vi "Functional acq video generator.vi"(7 "Channel":enum16{"Green", "Red"}(ring)=enum."Red", 9 "Input cluster":T2={"# of frames to export"=0, "Initial frame's owning file"=refnum, "8-bit AVI file path"=path "", "Cursors location"={"Number of first cycle"=0, "Number of last cycle"=100}}, 11 "ExperimentPath":path=path "C:/Users/Teo/Desktop/UCL Datasets/160915_13_48_57 FunctAcq-6 patches") -> ()   [LabVIEW 2020]
uses:
  Typedefs/Experiment Parameters.ctl
  Typedefs/Bright-Contr-Gamma cluster.ctl
  Timelapse Viewer/Typedefs/Speed graph behaviour enum.ctl
  <vilib>/vision/Avi.llb/IMAQ AVI2 Refnum.ctl
  Timelapse Viewer/Typedefs/8-bit video export window ctrl refs.ctl
  <vilib>/Utility/miscctls.llb/LVPointTypeDef.ctl
  Functional Imaging Viewer/Typedefs/Get-Set-Clear Control.ctl
  Timelapse Viewer/Globals/gl_Time series viewer globals.vi
  Globals/gl_8-bit montage window ctrl refs.vi
panel:
  in  "Speed graph behaviour":T3
  in  "Codec":u16(ring)=5 items=["No Codec", "Intel IYUV codec", "Cinepak Codec by Radius", "Microsoft Video 1", "FF Video Codec 1 (FFV1) (NI Vision)", "Motion JPEG (NI Vision)", "Y800 Uncompressed Grey Scale (NI Vision)", "YUV 4:2:0 Planar (NI Vision)"]
  in  "Microscope Image Adjustments":T4={"Brightness"=128.0, "Contrast"=45.0, "Gamma"=1.0} {"Gamma" min=0.5 scale=0.0..2.0; "Contrast" min=0.5 scale=0.0..90.0; "Brightness" min=0.5 scale=0.0..250.0}
  in  "Camera Video Adjustments":T4={"Brightness"=128.0, "Contrast"=45.0, "Gamma"=1.0} {"Gamma" min=0.5 scale=0.0..2.0; "Contrast" min=0.5 scale=0.0..90.0; "Brightness" min=0.5 scale=0.0..250.0}
  in  "Height of bottom tier":u32=120
  out "Frames Per Second":u32=26
  in  "Peak value in dataset (I16)":dbl=4000.0 format="%#_13g"
  in  "Number of rows to generate":i32=2
  in  "Execute":bool
  in  "Include speed graph":bool=TRUE
  in  "Include camera videos":bool
  in  "Enable saving":bool
  out "Image":T5(plugin-control)
  in  "Stop button":bool
  out "Global cycle number among all trials":i32 format="Current cycle: %.0f"
  out "Completion status":u8(slide) scale=0.0..100.0
  out "error out":errorcluster
  out "Experiment Parameters":T6
  out "Status":string
  # "This VI will be upgraded to handle volumetric data."
  # "<-- Adjusts the output dynamic range.\n       Temporary control."
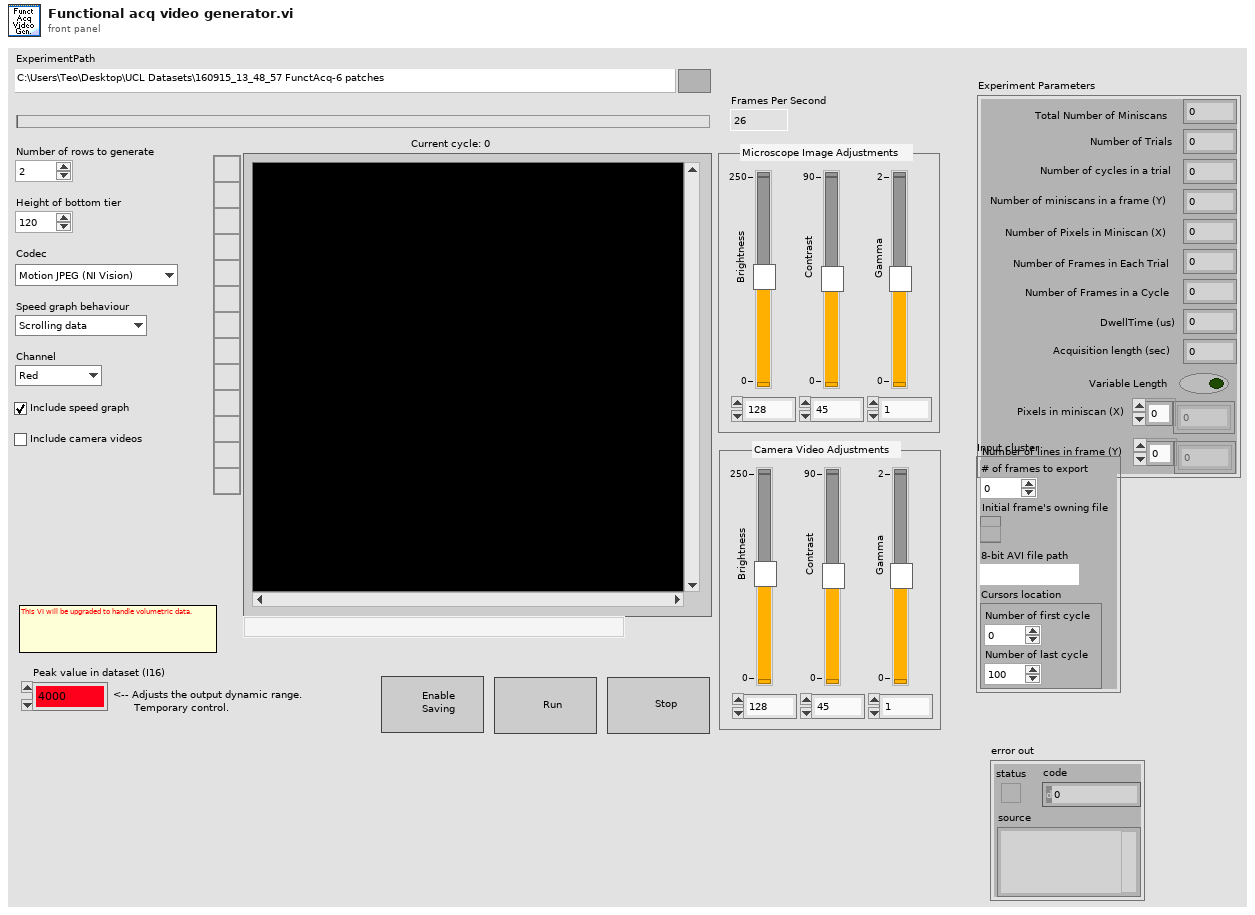
[diagram p1: front panel]
types:
  T1 = typedef "IMAQ AVI2 Refnum.ctl" = refnum<k20>
  T2 = cluster{"# of frames to export":i32, "Initial frame's owning file":T1, "8-bit AVI file path":path, "Cursors location":cluster{"Number of first cycle":i32, "Number of last cycle":i32}}
  T3 = typedef "Speed graph behaviour enum.ctl" = enum16{"Scrolling data", "Scrolling cursor"}
  T4 = typedef "Bright-Contr-Gamma cluster.ctl" = cluster{"Brightness":sgl, "Contrast":sgl, "Gamma":sgl}
  T5 = typedef "IMAQ Image.ctl" = refnum<image>
  T6 = typedef "Experiment Parameters.ctl" = cluster{"Total Number of Miniscans":i32, "Number of Trials":i32, "Number of cycles in a trial":i32, "Number of miniscans in a frame (Y)":i32, "Number of Pixels in Miniscan (X)":i32, "Number of Frames in Each Trial":i32, "Number of Frames in a Cycle":i32, "DwellTime (us)":dbl, "Acquisition length (sec)":dbl, "Variable Length":bool, "Pixels in miniscan (X)":dbl[], "Number of lines in frame (Y)":dbl[]}
  T7 = typedef "8-bit video export window ctrl refs.ctl" = cluster{"This VI":refnum<vi>, "Add speed data":refnum<vi>, "Add camera videos":refnum<vi>, "Stop button":refnum<vi>, "Camera Video Adjustments":refnum<vi>, "Microscope Image Adjustments":refnum<vi>, "Execute":refnum<vi>, "Codec":refnum<vi>, "Channel to load":refnum<vi>, "Speed graph behaviour":refnum<vi>, "Include speed graph":refnum<vi>, "Number of rows to generate":refnum<vi>, "Path":refnum<vi>}
  T8 = typedef "AVI playback header info cluster.ctl" = cluster{"Frame Size":u32, "AOD fill time (us)":dbl, "Dwell time (us)":dbl, "Frame period (ms)":dbl, "Number of Miniscans":u16, "Number of Pixels in Miniscan":u16}
  T9 = typedef "LVPointTypeDef.ctl" = cluster{"Horizontal":i16, "Vertical":i16}
  T10 = typedef "8bit sync-IMAQ image refs.ctl" = cluster{"Single patch (U8)":T5, "Adj.micr.bright & contrst (U8)":T5}
  T11 = typedef "Time series viewer refs.ctl" = cluster{"This VI":refnum<vi>, "Image control":refnum<vi>, "AVI Mode ind":refnum<vi>, "Play":refnum<vi>, "Stop":refnum<vi>, "Back":refnum<vi>, "Scrollbar":refnum<vi>, "Video length info":refnum<vi>, "Expected speed values":refnum<vi>, "Intensity":refnum<vi>, "Path":refnum<vi>, "Selection sliders":refnum<vi>, "Speed Graph ref":refnum<vi>, "Frame rate set (fps)":refnum<vi>, "Number of rows to generate":refnum<vi>, "VL Image Array":refnum<vi>, "Image Scrollbar":refnum<vi>, "Channel to load":refnum<vi>, "Colour":refnum<vi>}
  T12 = cluster{"Number of first cycle":i32, "Number of last cycle":i32}
  T13 = typedef "Get-Set-Clear Control.ctl" = enum16{"Get", "Set", "Clear"}
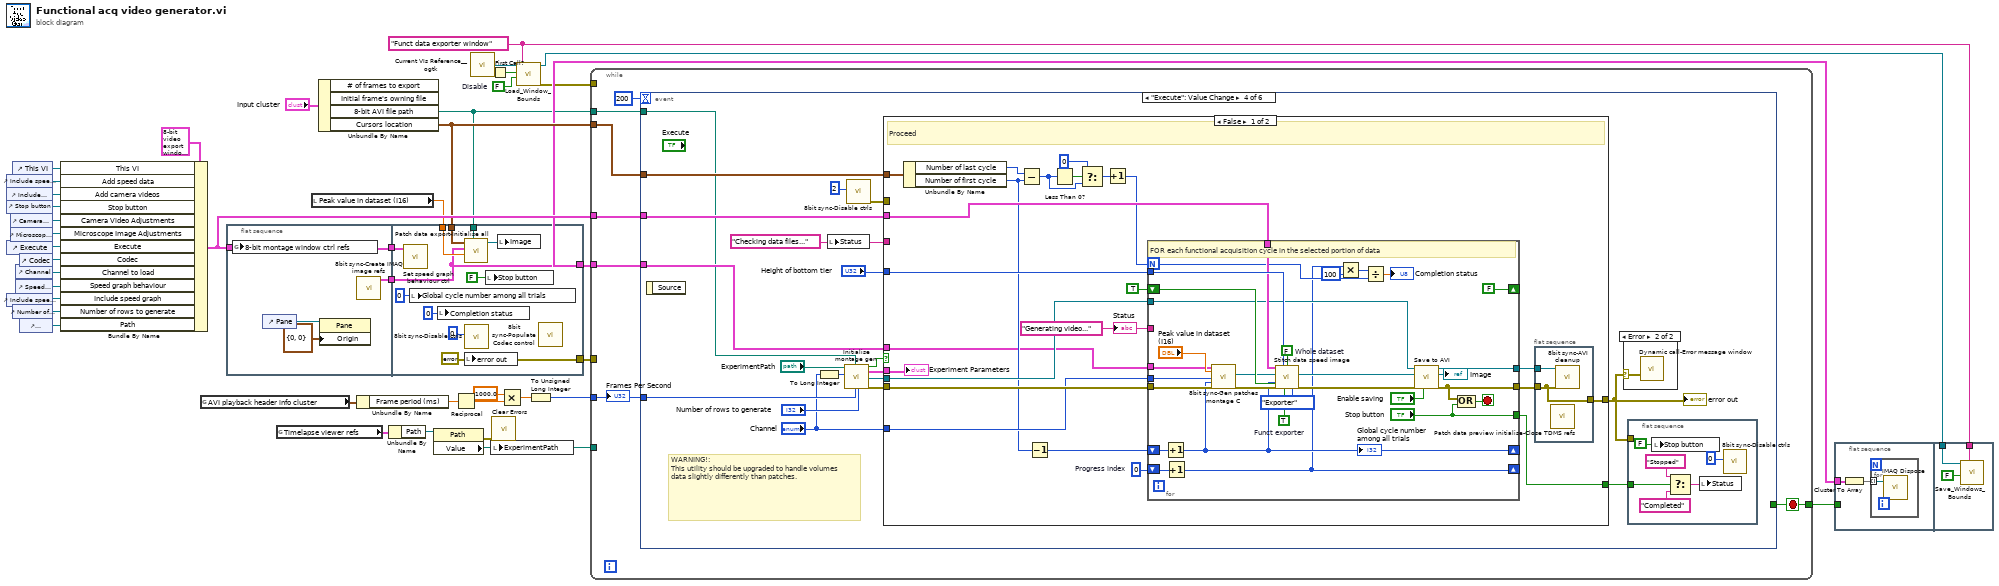
[diagram p0: block diagram]
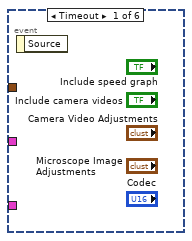
[diagram p2: hidden frame]
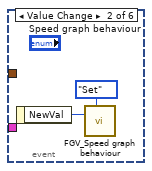
[diagram p3: hidden frame]
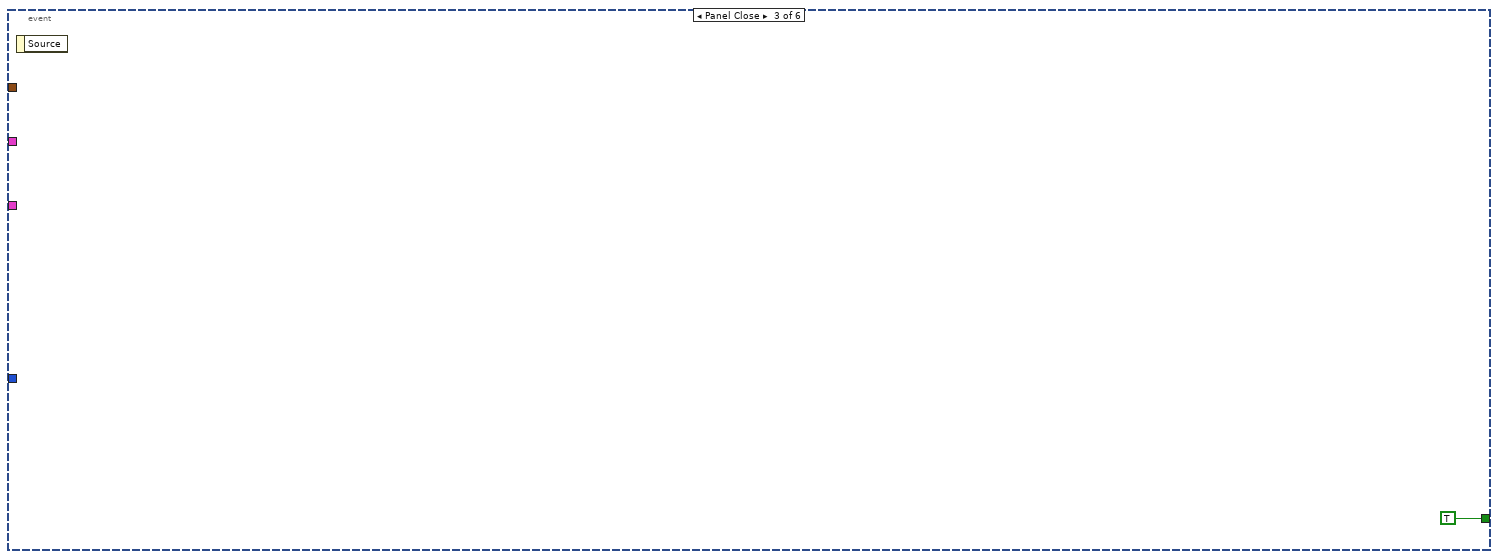
[diagram p4: hidden frame]
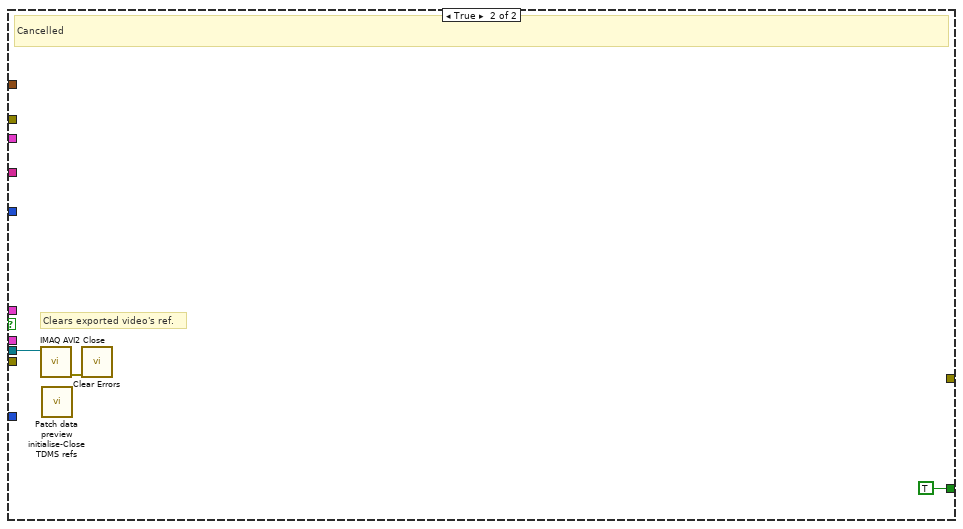
[diagram p6: hidden frame]
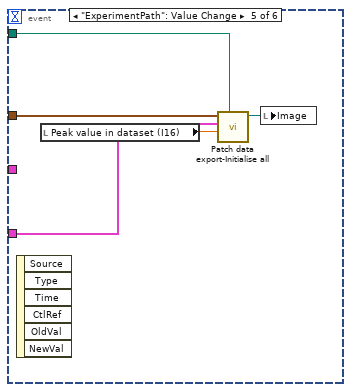
[diagram p7: hidden frame]
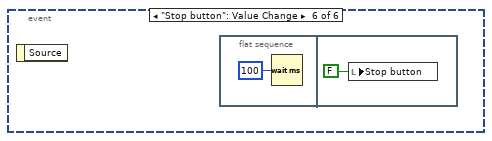
[diagram p8: hidden frame]
diagram:
  w4 = FALSE  # Disable
  w1 = "Funct data exporter window" ("Window Name (i.e. Key)")
  n1 = control-ref of="Include speed graph"() -> (w37:refnum<vi>)
  n2 = control-ref of="Include camera videos"() -> (w38:refnum<vi>)
  n3 = control-ref of="Stop button"() -> (w36:refnum<vi>)
  n4 = control-ref of="Execute"() -> (w33:refnum<vi>)
  n5 = control-ref of="Include speed graph"() -> (w18:refnum<vi>)
  n6 = control-ref of="Camera Video Adjustments"() -> (w35:refnum<vi>)
  n7 = control-ref of="Microscope Image Adjustments"() -> (w34:refnum<vi>)
  n8 = control-ref of="This VI"() -> (w12:refnum<vi>)
  n9 = control-ref of="Number of rows to generate"() -> (w17:refnum<vi>)
  n10 = control-ref of="Channel"() -> (w30:refnum<vi>)
  n11 = control-ref of="Speed graph behaviour"() -> (w23:refnum<vi>)
  n12 = control-ref of="Codec"() -> (w32:refnum<vi>)
  n13 = control-ref of="ExperimentPath"() -> (w16:refnum<vi>)
  n14 = Bundle By Name(cluster=T7 {"This VI"=refnum, "Add speed data"=refnum, "Add camera videos"=refnum, "Stop button"=refnum, "Camera Video Adjustments"=refnum, "Microscope Image Adjustments"=refnum, "Execute"=refnum, "Codec"=refnum, "Channel to load"=refnum, "Speed graph behaviour"=refnum, "Include speed graph"=refnum, "Number of rows to generate"=refnum, "Path"=refnum} ("output cluster"), "This VI"=w12, "Add speed data"=w37, "Add camera videos"=w38, "Stop button"=w36, "Camera Video Adjustments"=w35, "Microscope Image Adjustments"=w34, "Execute"=w33, "Codec"=w32, "Channel to load"=w30, "Speed graph behaviour"=w23, "Include speed graph"=w18, "Number of rows to generate"=w17, "Path"=w16) -> (w31:T7)
  n15 = global read "gl_Time series viewer globals.vi" "AVI playback header info cluster"() -> (w29:T8)
  n16 = flat-sequence {
    tunnel: w31 -> [w44]
    tunnel: [w44] -> w15
    tunnel: [w43] -> w11
    tunnel: [w53] -> w40
    tunnel: w15 -> [w50]
    tunnel: w14 -> [w49]
    tunnel: w13 -> [w47]
    tunnel: w11 -> [w46]
    tunnel: [w46] -> w9
    tunnel: w8 -> [w45]
    frame #0 {
      n17 = global write "gl_8-bit montage window ctrl refs.vi" "8-bit montage window ctrl refs"(w44) -> ()
      n18 = control-ref of="Pane"() -> (w41:refnum<vi>)
      n19 = property class="Pane"(reference=w41, "Origin"=T9 {"Horizontal"=0, "Vertical"=0}) -> ()  [unwired: 1 in, 2 out]
      n20 = call "8bit sync-Create IMAQ image refs.vi"() -> ("8-bit Image refs cluster"=w43:T10)  [unwired: 11 in]
    }
    frame #1 {
      w53 = errorcluster {"status"=FALSE, "code"=0, "source"=""} ("error in (no error)")
      n21 = call "Set speed graph behaviour ctrl.vi"("Exporter's ctrl refs"=w50) -> ()  [unwired: 10 in, 1 out]
      n22 = local write "Global cycle number among all trials"(0 ("Frames written")) -> ()
      n23 = local write "Completion status"(u8 0 ("Slide")) -> ()
      n24 = call "Patch data export-Initialise all.vi"("Output file path"=w45, "Peak value in dataset (I16)"=w47, "8-bit Image refs cluster"=w46, "Cursors location"=w49) -> ("U8 Image ref"=w48:T5)  [unwired: 6 in, 1 out]
      n25 = local write "error out"(w53) -> ()
      n26 = call "8bit sync-Disable ctrls.vi"("Disabled"=0) -> ()  [unwired: 10 in, 1 out]
      n27 = local write "Stop button"(FALSE ("Stop")) -> ()
      n28 = local write "Image"(w48) -> ()
      n29 = call "8bit sync-Populate Codec control.vi"() -> ()  [unwired: 11 in, 1 out]
    }
  }
  n30 = global read "gl_Time series viewer globals.vi" "Timelapse viewer refs"() -> (w21:T11)
  n31 = local read "Peak value in dataset (I16)"() -> (w13:dbl)
  n32 = Unbundle By Name("Input cluster") -> ("8-bit AVI file path"=w8:path, "Cursors location"=w14:T12)  [unwired: 2 out]
  n33 = Unbundle By Name(w29) -> ("Frame period (ms)"=w28:dbl)
  n34 = Unbundle By Name(w21) -> ("Path"=w20:refnum<vi>)
  n35 = property class="Path"(reference=w20) -> (error out=w7:errorcluster, "Value"=w19:path)  [unwired: 1 in, 1 out]
  n36 = Reciprocal(x=w28) -> (1/x=w26:dbl)
  n37 = call <userlib>:"Current VIs Reference__ogtk.vi"() -> ("Current VI's reference"=w6:refnum<vi>)  [unwired: 5 in]
  n38 = First Call?() -> (First Call?: T/F=w5:bool)
  n39 = local write "ExperimentPath"(w19) -> ()
  n40 = call <vilib>:"Clear Errors.vi"("error in (no error)"=w7) -> ()  [unwired: 5 in, 2 out]
  n41 = Multiply(x=1000.0, y=w26) -> (x*y=w25:dbl)
  n42 = call "Load_Window_Bounds.vi"("Window Name (i.e. Key)"=w1, "Disable"=w4, "First Call"=w5, "Window VI's Ref"=w6) -> ("error out"=w3:errorcluster, "reference out"=w2:refnum<vi>)  [unwired: 4 in, 2 out]
  n43 = To Unsigned Long Integer(number=w25) -> (unsigned 32bit integer=w27:u32)
  n44 = while {
    tunnel: w40 -> [_]
    tunnel: w31 -> [w61]
    tunnel: w27 -> [w60]
    tunnel: w14 -> [w59]
    tunnel: w19 -> [_]
    tunnel: w9 -> [w58]
    tunnel: [w57] -> w10
    tunnel: w8 -> [w56]
    tunnel: w3 -> [_]
    stop <- w57 stop-if-true
    n45 = event shown="[3] \"Execute\": Value Change" {
      selector: _ -> [_ _ _ _ _ _]
      dyn-events: _ -> [_ _ _ _ _ _]
      timeout: 200 -> [_ _ _ _ _ _]
      tunnel: [_ _ TRUE _ _ _] -> w57
      tunnel: w61 -> [_ _ _ w80 _ _]
      tunnel: w60 -> [_ _ _ w76 _ _]
      tunnel: w59 -> [_ _ _ w75 w153 _]
      tunnel: w58 -> [_ _ _ w67 w151 _]
      tunnel: w56 -> [_ _ _ w66 w150 _]
      event Timeout {
        n46 = event-data() -> ()  [unwired: 1 in, 1 out]
      }
      event Value Change {
        n47 = event-data() -> ("NewVal"=w63:T3)  [unwired: 1 in]
        n48 = call "FGV_Speed graph behaviour.vi"("Function"=Get-Set-Clear_Control."Set", "Speed graph behaviour"=w63) -> ()  [unwired: 8 in, 2 out]
      }
      event Panel Close {
        n49 = event-data() -> ()  [unwired: 1 in, 1 out]
      }
      event "Execute": Value Change {
        w83 = "Checking data files..." ("Status")
        # "WARNING!:\nThis utility should be upgraded to handle volumes data slightly differently than patches."
        n50 = event-data() -> ()  [unwired: 1 in, 1 out]
        n51 = To Long Integer(number="Channel") -> (32bit integer=w68:i32)
        n52 = local write "Status"(w83) -> ()
        n53 = call "Initialise montage gen.vi"("ExperimentPath"="ExperimentPath", "Channel"=w68, "Output file path"=w66, "Frames Per Second"=w76, "Number of rows to generate"="Number of rows to generate") -> ("Cancel"=w71:bool, "Experiment Parameters"=w70:T6, "Output file ref"=w72:T1, "error out"=w84:errorcluster)  [unwired: 11 in]
        n54 = call "8bit sync-Disable ctrls.vi"("Disabled"=2) -> ("error out"=w78:errorcluster)  [unwired: 10 in]
        n55 = case shown="False" w71 {
          tunnel: w70 -> [w108 _]
          tunnel: w84 -> [w113 _]
          tunnel: [w114 _] -> w81
          tunnel: w83 -> [_ _]
          tunnel: [w112 TRUE ("Stop")] -> w82
          tunnel: w80 -> [w109 _]
          tunnel: "Height of bottom tier" -> [w110 _]
          tunnel: w78 -> [_ _]
          tunnel: "Channel" -> [w103 _]
          tunnel: w75 -> [w102 _]
          tunnel: w72 -> [w100 w147]
          tunnel: w67 -> [w96 _]
          frame False {
            w104 = "Generating video..." ("Status")
            w107 = 0  # Progress index
            # "Proceed"
            n56 = Unbundle By Name(w102) -> ("Number of last cycle"=w101:i32, "Number of first cycle"=w97:i32)
            n57 = Subtract(x=w101, y=w97) -> (x-y=w94:i32)
            n58 = Decrement(x=w97) -> (x-1=w95:i32)
            n59 = Less Than 0?(x=w94) -> (x < 0?=w99:bool)
            n60 = Select(t=0, s=w99, f=w94) -> (s? t:f=w93:i32)
            n61 = Increment(x=w93) -> (x+1=w92:i32)
            n62 = for {
              N: w92 -> [w127]
              tunnel: w100 -> [w128]
              tunnel: [w142] -> w106
              tunnel: [w137] -> w105
              tunnel: w113 -> [w146]
              shift-right: [w126] -> _
              shift-left: w95 -> [w138]
              tunnel: ["Stop button"] -> w112
              shift-right: [FALSE] -> _
              shift-left: TRUE -> [w134]
              tunnel: w109 -> [w133]
              tunnel: w110 -> [w139]
              shift-right: [w124] -> _
              shift-left: w107 -> [w125]
              tunnel: w104 -> [_]
              tunnel: w103 -> [w121]
              tunnel: w96 -> [w118]
              stop <- w141 stop-if-true
              w123 = FALSE  # Whole dataset
              w130 = TRUE  # Funct exporter
              # "FOR each functional acquisition cycle in the selected portion of data"
              n63 = Increment(x=w138) -> (x+1=w126:i32)
              "Global cycle number among all trials" <- w126
              n64 = Increment(x=w125) -> (x+1=w124:i32)
              n65 = call "8bit sync-Gen patches montage C.vi"("8-bit Image refs cluster"=w118, "max value"="Peak value in dataset (I16)", "Channel"=w121, "Global cycle number among all trials"=w126, "error in (no error)"=w146) -> ("U8 Image (Montage)"=w120:T5, "error out"=w135:errorcluster)  [unwired: 13 in]
              n66 = call "Stitch data speed image.vi"("Ctrl refs"=w133, "Required Y-axis size of bottom tier"=w139, "Whole dataset"=w123, "Caller"=enum16{"Viewer", "Exporter"}."Exporter", "Microscope image"=w120, "Global frame number in master video(s)"=w126, "error in (no error)"=w135, "Initial frame"=w134, "Funct exporter"=w130) -> ("Stitched Image"=w131:T5, "error out"=w136:errorcluster)  [unwired: 5 in]
              n67 = Multiply(x=w124, y=100) -> (x*y=w144:i32)
              n68 = Divide(x=w144, y=w127) -> (x/y=→"Completion status":dbl)
              n69 = call "Save to AVI.vi"("Enable saving"="Enable saving", "error in (no error)"=w136, "Refnum in"=w131, "AVI Refnum"=w128) -> ("error out"=w142:errorcluster, "Refnum out"=→"Image":T5, "AVI Refnum (duplicate)"=w137:T1)  [unwired: 5 in]
              n70 = Compound Arithmetic op=OR(w142, "Stop button") -> (w141:bool)
            }
            n71 = flat-sequence {
              tunnel: [w115] -> w114
              tunnel: w106 -> [w115]
              tunnel: w105 -> [w116]
              frame #0 {
                n72 = call "Patch data preview initialise-Close TDMS refs.vi"() -> ()  [unwired: 11 in, 1 out]
                n73 = call "8bit sync-AVI cleanup.vi"("error in (no error)"=w115, "Output AVI ref"=w116) -> ()  [unwired: 10 in]
              }
            }
            "Experiment Parameters" <- w108
            "Status" <- w104
          }
          frame True {
            # "Clears exported video's ref."
            # "Cancelled"
            n74 = call "IMAQ AVI2 Close"("AVI Refnum"=w147) -> ("error out"=w149:errorcluster)  [unwired: 10 in]
            n75 = call "Patch data preview initialise-Close TDMS refs.vi"() -> ()  [unwired: 11 in, 1 out]
            n76 = call <vilib>:"Clear Errors.vi"("error in (no error)"=w149) -> ()  [unwired: 5 in, 2 out]
          }
        }
        "error out" <- w81
        n77 = case shown="Error" w81 {
          selector: w81 -> [_ w85]
          frame No Error {
          }
          frame Error {
            n78 = call "Dynamic call-Error message window.vi"("error in (no error)"=w85) -> ()  [unwired: 10 in, 1 out]
          }
        }
        n79 = flat-sequence {
          tunnel: w81 -> [_]
          tunnel: w82 -> [w87]
          frame #0 {
            n80 = local write "Stop button"(FALSE ("Stop")) -> ()
            n81 = Select(t="Stopped" ("Status"), s=w87, f="Completed" ("Status")) -> (s? t:f=w88:string)
            n82 = local write "Status"(w88) -> ()
            n83 = call "8bit sync-Disable ctrls.vi"("Disabled"=0) -> ()  [unwired: 10 in, 1 out]
          }
        }
      }
      event "ExperimentPath": Value Change {
        n84 = event-data() -> ()  [unwired: 1 in, 6 out]
        n85 = local read "Peak value in dataset (I16)"() -> (w152:dbl)
        n86 = call "Patch data export-Initialise all.vi"("Output file path"=w150, "Peak value in dataset (I16)"=w152, "8-bit Image refs cluster"=w151, "Cursors location"=w153) -> ("U8 Image ref"=w154:T5)  [unwired: 6 in, 1 out]
        n87 = local write "Image"(w154) -> ()
      }
      event "Stop button": Value Change {
        n88 = event-data() -> ()  [unwired: 1 in, 1 out]
        n89 = flat-sequence {
          frame #0 {
            n90 = Wait (ms)(milliseconds to wait=u32 100) -> ()  [unwired: 1 out]
          }
          frame #1 {
            n91 = local write "Stop button"(FALSE ("Stop")) -> ()
          }
        }
      }
    }
    "Frames Per Second" <- w60
  }
  n92 = flat-sequence {
    tunnel: w9 -> [w158]
    tunnel: w10 -> [_]
    tunnel: w2 -> [w162]
    tunnel: w1 -> [w160]
    frame #0 {
      n93 = Cluster To Array(cluster=w158) -> (array=w157:T5[])
      n94 = for {
        tunnel: w157 -> [w159] mode=indexing
        n95 = call "IMAQ Dispose"("Image"=w159) -> ()  [unwired: 5 in, 1 out]
      }
    }
    frame #1 {
      n96 = call "Save_Windows_Bounds.vi"("Window Name (i.e. Key)"=w160, "Front Panel Window:Open"=FALSE, "Window VI's Ref"=w162) -> ()  [unwired: 8 in, 1 out]
    }
  }
